vi "BatterySim_CalculateLoadedBatteryVoltage.vi"(9 "Currents":dbl[](array[numeric]), 10 "Resistance_Ohms":dbl, 11 "NominalVoltage":dbl) -> (3 "Voltage":dbl)   [LabVIEW 2019, in "Trajectory_Library.lvlib"]
doc: "Utility function to calculate distance (hypotenuse) result = ( x ^2 + y ^2 ) ^ 0.5\n\nParameters:\n - X\n - Y\n\nResult\n - Distance"
uses:
  Trajectory_Library.lvlib
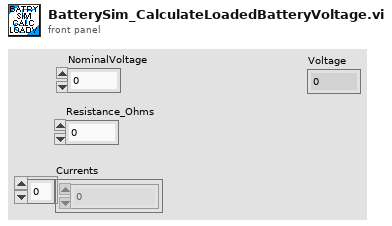
[diagram p1: front panel]
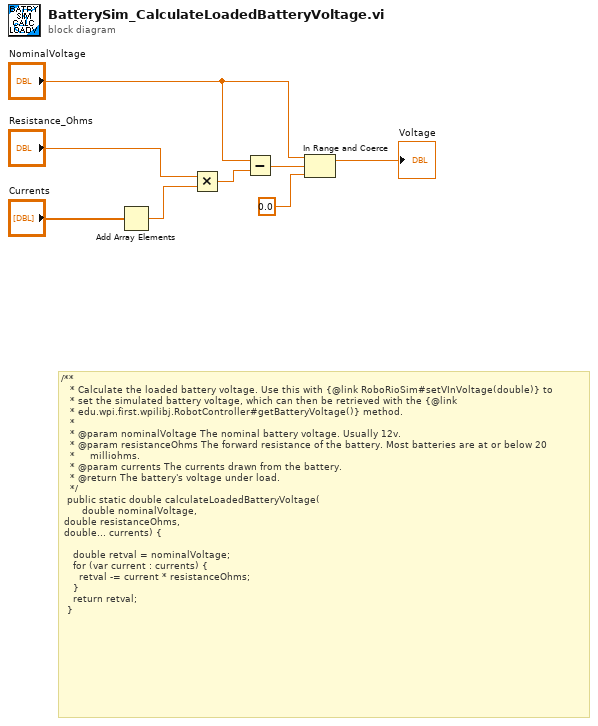
[diagram p0: block diagram]
diagram:
  # "/**\n   * Calculate the loaded battery voltage. Use this with {@link RoboRioSim#setVInVoltage(double)} to\n   * set the simulated battery voltage, which can then be retrieved with the {@link\n   * edu.wpi.first.wpilibj.RobotController#getBatteryVoltage()} method.\n   *\n   * @param nominalVoltage The nominal battery voltage. Usually 12v.\n   * @param resistanceOhms The forward resistance of the battery. Most batteries are at or below 20\n   *     milliohms.\n   * @param currents The currents drawn from the battery.\n   * @return The battery's voltage under load.\n   */\n  public static double calculateLoadedBatteryVoltage(\n      \tdouble nominalVoltage, \n\tdouble resistanceOhms, \n\tdouble... currents) {\n\n    double retval = nominalVoltage;\n    for (var current : currents) {\n      retval -= current * resistanceOhms;\n    }\n    return retval;\n  }"
  n1 = Add Array Elements(numeric array="Currents") -> (sum=w6:dbl)
  n2 = Multiply(x="Resistance_Ohms", y=w6) -> (x*y=w2:dbl)
  n3 = Subtract(x="NominalVoltage", y=w2) -> (x-y=w3:dbl)
  n4 = In Range and Coerce(upper limit="NominalVoltage", x=w3, lower limit=0.0) -> (coerced(x)=→"Voltage":dbl)  [unwired: 1 out]
